vi "Name.vi"(1 "Hash Function in":refnum<class "NI_SHA-3.lvclass">) -> (0 "String":string)   [LabVIEW 2020, in "NI_SHA-3.lvclass"]
uses:
  <vilib>/security/Message Digest/SHA-3/NI_SHA-3.lvclass
  <vilib>/security/Message Digest/SHA-3/NI_SHA-3.lvclass/NI_SHA-3.ctl
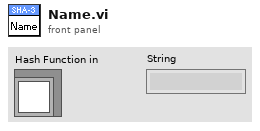
[diagram p1: front panel]
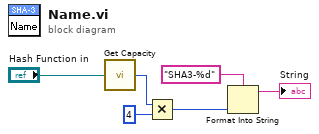
[diagram p0: block diagram]
diagram:
  n1 = call <vilib>:"Get Capacity.vi"("Hash Function in"="Hash Function in") -> ("capacity"=w2:i32)
  n2 = Multiply(x=w2, y=4) -> (x*y=w5:i32)
  n3 = Format Into String(format string="SHA3-%d", w5) -> (resulting string=→"String":string)  [unwired: 2 in, 1 out]
